vi "Cluster.vi"(8 "Error In":errorcluster) -> (0 "Error Out":errorcluster)   [LabVIEW 2018, in "Tests.lvlib" / "From Msgpack.lvlib"]
uses:
  From Msgpack.lvlib
  <vilib>/addons/_JKI Toolkits/Caraya/classes/Test/Test.lvclass
  src/LabPack/Toolkit.lvlib
  <vilib>/addons/_JKI Toolkits/Caraya/classes/Assert/Assert.lvclass
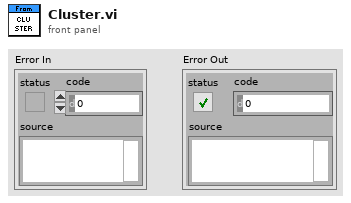
[diagram p1: front panel]
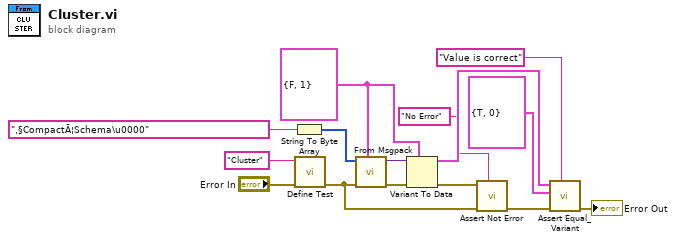
[diagram p0: block diagram]
diagram:
  w2 = cluster{"Compact":bool, "Schema":i32} {"Compact"=FALSE, "Schema"=1}
  n1 = String To Byte Array(string="‚§CompactÃ¦Schema\u0000") -> (unsigned byte array=w12:u8[])
  n2 = call <vilib>:"Define Test.vi"("error in (no error)"="Error In", "Label (VI Title)"="Cluster") -> ("error out"=w9:errorcluster)  [unwired: 9 in]
  n3 = call "From Msgpack.vi"("Types and Defaults"=w2, "Error In"=w9, "Msgpack Data"=w12) -> ("Error Out"=w13:errorcluster, "Value"=w11:variant)  [unwired: 7 in]
  n4 = Variant To Data(error in=w13, type=w2, Variant=w11) -> (data=w6:cluster{"Compact":bool, "Schema":i32}, error out=w10:errorcluster)
  n5 = call <vilib>:"Assert Not Error.vi"("Label"="No Error", "error in (no error)"=w9, "Not Error?"=w10) -> ("error out"=w8:errorcluster)  [unwired: 8 in]
  n6 = call <vilib>:"Assert Equal_Variant.vi"("Label"="Value is correct", "error in (no error)"=w8, "Y"=cluster{"Compact":bool, "Schema":i32} {"Compact"=TRUE, "Schema"=0}, "X"=w6) -> ("error out"=→"Error Out":errorcluster)  [unwired: 7 in]
